vi "GetFlattenedString.vi"(8 "error in":errorcluster, 11 "Int in":refnum<class "Int.lvclass">) -> (0 "error out":errorcluster, 2 "FlattenedString":string, 3 "Int out":refnum<class "Int.lvclass">)   [LabVIEW 2021, in "ProligentXMLGenerator.lvlib" / "Int.lvclass"]
uses:
  Int.lvclass
  Int.lvclass/Int.ctl
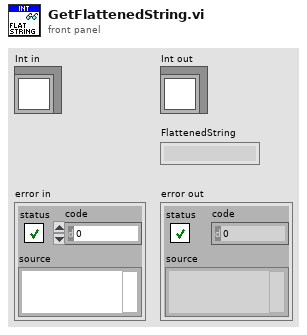
[diagram p1: front panel]
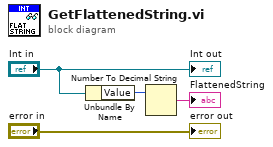
[diagram p0: block diagram]
diagram:
  n1 = Unbundle By Name("Int in") -> ("Value"=w2:i32)
  n2 = Number To Decimal String(number=w2) -> (decimal integer string=→"FlattenedString":string)  [unwired: 1 in]
  "error out" <- "error in"
  "Int out" <- "Int in"
